vi "fix documentation.vi"() -> ()   [LabVIEW 2023]
uses:
  <vilib>/xml/Close Reference(Node).vi
  <vilib>/xml/NI_XML.lvlib
  <resource>/objmgr/DOMUserDefRef.rc
panel:
  out "Numeric":i32
  out "Array":cluster{"Name":string, "Name":string}[](array[cluster])
  out "error out":errorcluster
  out "XML":string
  out "Parse Errors":string
  in  "XML File Path":path
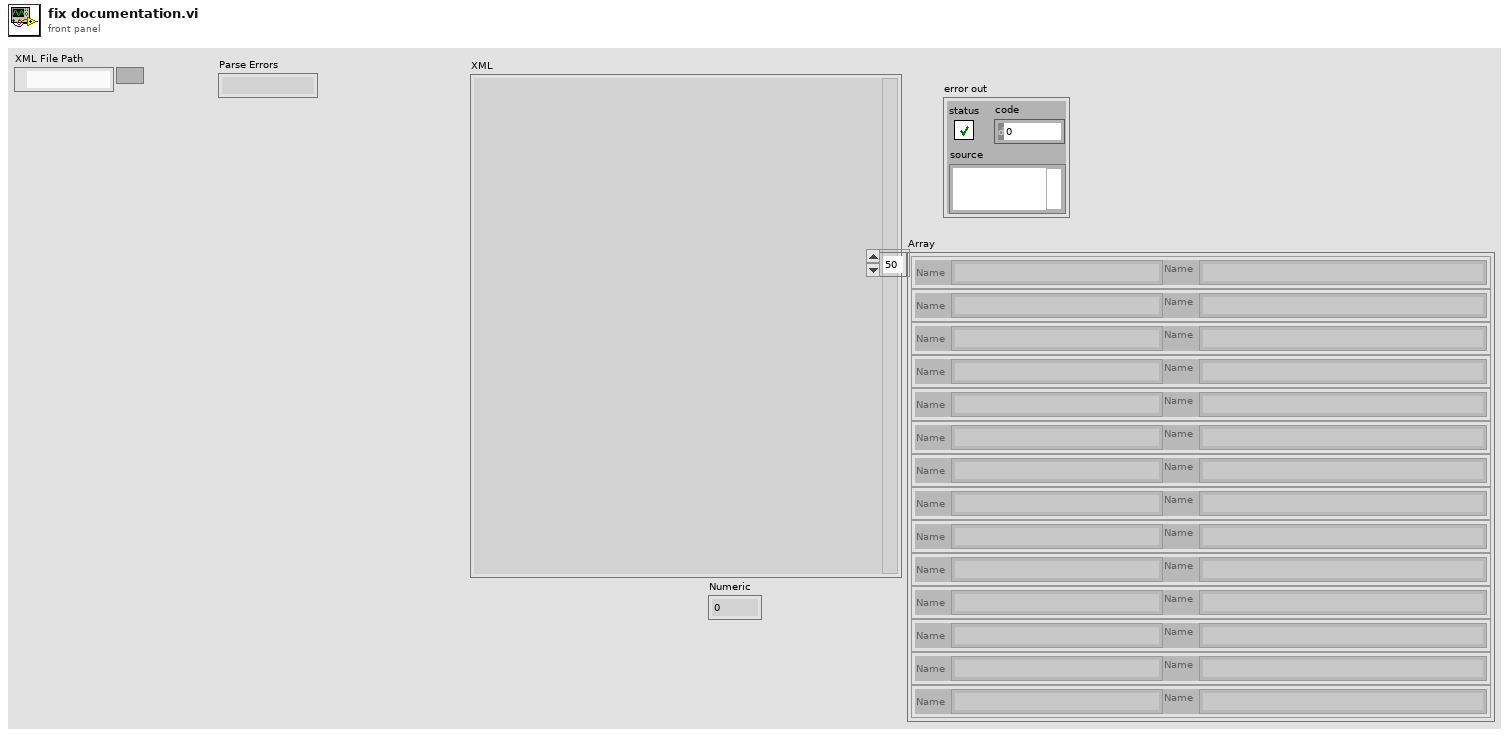
[diagram p1: front panel]
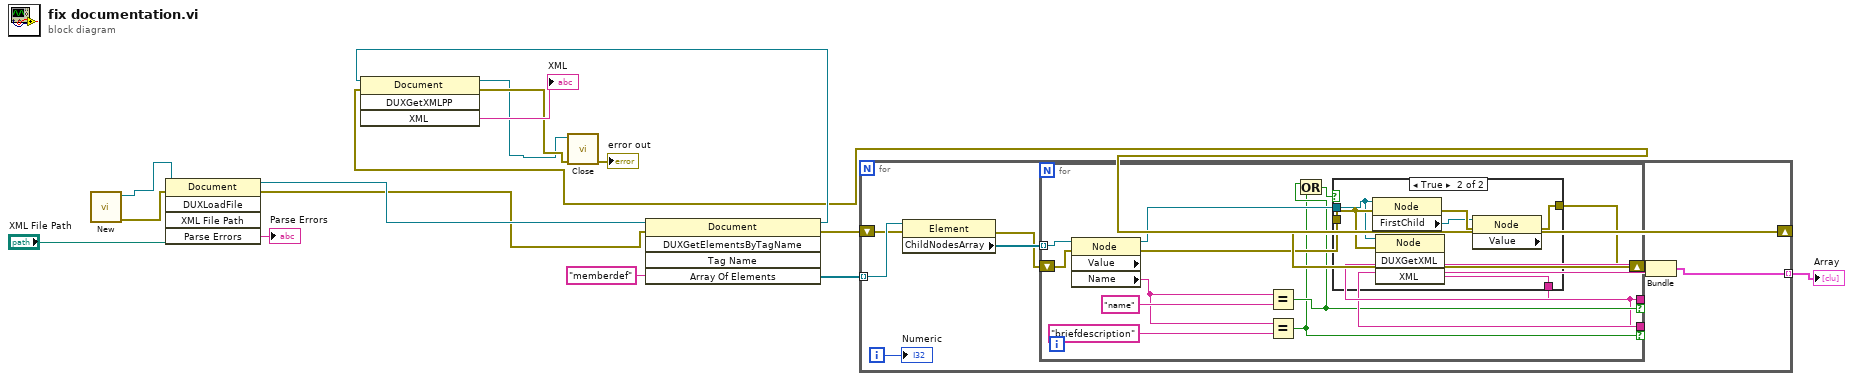
[diagram p0: block diagram]
diagram:
  n1 = call <vilib>:"New.vi"() -> ("error out"=w13:errorcluster, "DOM document out"=w16:refnum<k20>)  [unwired: 8 in]
  n2 = invoke class="Document" method="DUXLoadFile"(reference=w16, error in=w13, "XML File Path"="XML File Path") -> (reference out=w3:refnum<k20>, error out=w1:errorcluster, "Parse Errors"=→"Parse Errors":string)  [unwired: 2 in, 2 out]
  n3 = invoke class="Document" method="DUXGetElementsByTagName"(reference=w3, error in=w1, "Tag Name"="memberdef") -> (reference out=w6:refnum<k20>, error out=w8:errorcluster, "Array Of Elements"=w9:refnum<k20>[])  [unwired: 2 in, 2 out]
  n4 = for {
    tunnel: w9 -> [w25] mode=indexing
    shift-right: [w21] -> w5
    shift-left: w8 -> [w24]
    tunnel: [w18] -> w7 mode=indexing
    i -> [w17]
    n5 = property class="Element"(reference=w25, error in=w24) -> (error out=w22:errorcluster, "ChildNodesArray"=w23:refnum<k20>[])  [unwired: 1 out]
    n6 = for {
      tunnel: w23 -> [w37] mode=indexing
      shift-right: [w30] -> w21
      shift-left: w22 -> [w36]
      tunnel: [w26] -> w20 if=w29
      tunnel: [w26] -> w19 if=w27
      n7 = property class="Node" props=["Value", "Name"](reference=w37, error in=w36) -> (reference out=w32:refnum<k20>, error out=w31:errorcluster, "Name"=w33:string)  [unwired: 1 out]
      n8 = Equal?(x=w33, y="name") -> (x = y?=w29:bool)
      n9 = Equal?(x=w33, y="briefdescription") -> (x = y?=w27:bool)
      n10 = Or(x=w29, y=w27) -> (x .or. y?=w28:bool)
      n11 = case shown="True" w28 {
        tunnel: w32 -> [_ w39]
        tunnel: w31 -> [w38 w42]
        tunnel: [w38 w43] -> w30
        tunnel: [_ w41] -> w26
        frame False {
        }
        frame True {
          n12 = property class="Node"(reference=w39, error in=w42) -> (error out=w44:errorcluster, "FirstChild"=w40:refnum<k20>)  [unwired: 1 out]
          n13 = invoke class="Node" method="DUXGetXML"(reference=w39, error in=w42) -> ("XML"=w41:string)  [unwired: 2 in, 3 out]
          n14 = property class="Node" props=["Value"](reference=w40, error in=w44) -> (error out=w43:errorcluster)  [unwired: 2 out]
        }
      }
    }
    n15 = Bundle("XML"=w20, "XML"=w19) -> (w18:cluster{"XML":string, "XML":string})  [unwired: 1 in]
    "Numeric" <- w17
  }
  "Array" <- w7
  n16 = invoke class="Document" method="DUXGetXMLPP"(reference=w6, error in=w5) -> (reference out=w2:refnum<k20>, error out=w4:errorcluster, "XML"=→"XML":string)  [unwired: 2 in, 1 out]
  n17 = call-poly <vilib>:"Close.vi"("error in (no error)"=w4, "node"=w2) -> ("error out"=→"error out":errorcluster)  [unwired: 7 in]
